vi "Generare_numar_aleator.vi"() -> ()   [LabVIEW 2019]
uses:
  <vilib>/numeric/Random Number (Range) DBL.vi
panel:
  out "Afisare numar aleator 2":dbl(graph)
  in  "Numar 2":dbl
  out "Afisare numar aleator":dbl(graph)
  in  "Numar":dbl
  # "Generare numar aleator"
  # "Dorim sa generam un\n numar cuprins intre:"
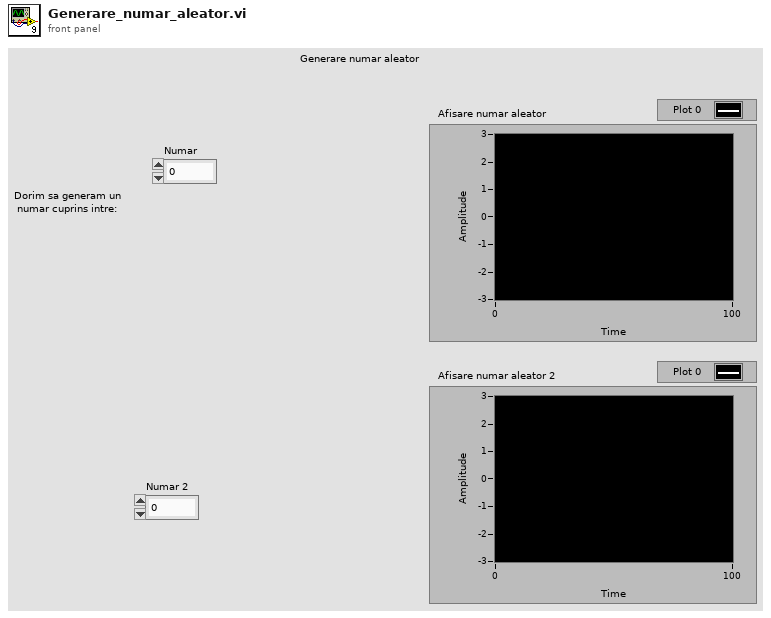
[diagram p1: front panel]
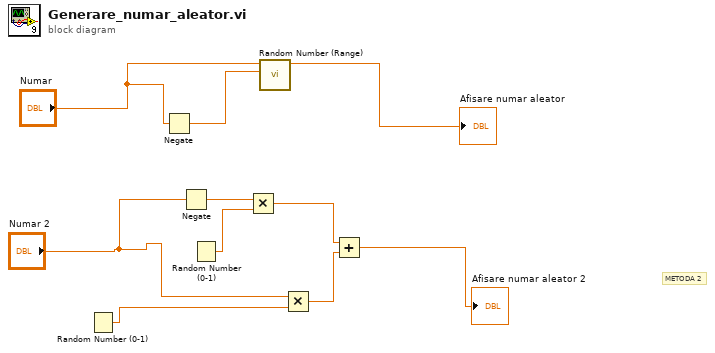
[diagram p0: block diagram]
diagram:
  # "METODA 2"
  n1 = Random Number (0-1)() -> (number: 0 to 1=w7:dbl)
  n2 = Negate(x="Numar") -> (-x=w9:dbl)
  n3 = Negate(x="Numar 2") -> (-x=w5:dbl)
  n4 = Random Number (0-1)() -> (number: 0 to 1=w4:dbl)
  n5 = Multiply(x=w5, y=w4) -> (x*y=w3:dbl)
  n6 = call-poly <vilib>:"Random Number (Range).vi"("lower bound (0)"=w9, "upper bound (100)"="Numar") -> ("number"=→"Afisare numar aleator":dbl)  [unwired: 9 in]
  n7 = Multiply(x="Numar 2", y=w7) -> (x*y=w2:dbl)
  n8 = Add(x=w3, y=w2) -> (x+y=→"Afisare numar aleator 2":dbl)
